vi "Open.vi"(8 "error in (no error)":errorcluster) -> (0 "error out":errorcluster, 3 "FPGA Refs":T1)   [LabVIEW 2017, in "Piezo Controller.lvlib"]
uses:
  Piezo Controller.lvlib
  FPGA Refs.ctl
  <instrlib>/_niInstr/FIFO Register Bus/v1/Host/niInstr FIFO Register Bus v1 Host.lvclass
  C:/Program Files (x86)/National Instruments/LabVIEW 2017/instr.lib/_niInstr/Instruction Framework/v1/Host/Instruction Target/niInstr Instruction Target v1 Host.lvclass
  <instrlib>/_niInstr/Instruction Framework/v1/Host/Instruction Framework Context/niInstr Instruction Framework Context v1 Host.lvclass
  <vilib>/FPGAPlugInAG/PCIe-7852R/niLvFpga_Open_PCIe-7852R.vi
  <vilib>/rvi/interface/common/dynamic/niFpgaDynamicAddResources.vi
  <instrlib>/_niInstr/Instruction Framework/v1/Host/Subsystem Map/Private/Lookup Single Context.vi
  <vilib>/rvi/interface/nirviOpenFPGA/nirviOpenFPGA.xnode
  Builds/Bitfile/vibratome_single_channel.lvbitx
  <instrlib>/_niInstr/Instruction Framework/v1/Host/Subsystem Map/niInstr Subsystem Map v1 Host.lvclass
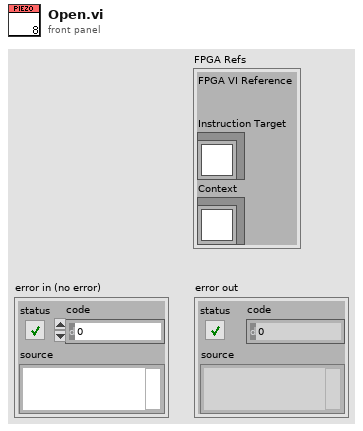
[diagram p1: front panel]
types:
  T1 = typedef "Piezo Controller.lvlib/FPGA Refs.ctl" = cluster{"FPGA VI Reference":refnum<k20>, "Instruction Target":refnum<class "niInstr FIFO Register Bus v1 Host.lvclass">, "Context":refnum<class "niInstr Instruction Framework Context v1 Host.lvclass">}
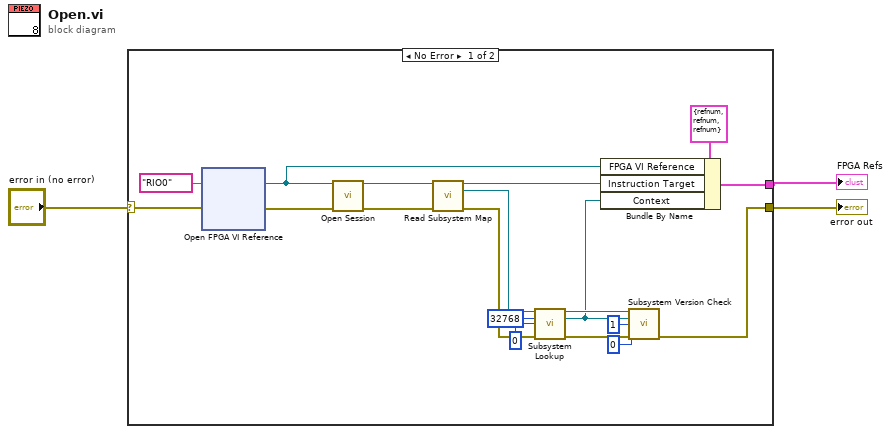
[diagram p0: block diagram]
diagram:
  n1 = case shown="No Error" "error in (no error)" {
    selector: "error in (no error)" -> [w5 w23]
    tunnel: [w6 _] -> w1
    tunnel: [w4 w23] -> w2
    frame No Error {
      n2 = xnode "Open FPGA VI Reference"("error in"=w5, "resource name"=tag "RIO0") -> ("FPGA VI Reference Out"=w10:refnum<k20>, "error out"=w22:errorcluster)
      n3 = call <instrlib>:"Open Session.vi"("fpga ref"=w10, "error in"=w22) -> ("session out"=w20:refnum<class "niInstr FIFO Register Bus v1 Host.lvclass">, "error out"=w21:errorcluster)  [unwired: 12 in]
      n4 = call <instrlib>:"Read Subsystem Map.vi"("instruction target in"=w20, "error in"=w21) -> ("instruction target out"=w9:refnum<class "niInstr FIFO Register Bus v1 Host.lvclass">, "subsystem map"=w14:refnum<class "niInstr Subsystem Map v1 Host.lvclass">, "error out"=w19:errorcluster)  [unwired: 11 in]
      n5 = call-poly <instrlib>:"Subsystem Lookup.vi"("subsystem map in"=w14, "UID"=u16 32768, "instance"=u8 0, "error in"=w19) -> ("subsystem map out"=w17:refnum<class "niInstr Subsystem Map v1 Host.lvclass">, "context"=w8:refnum<class "niInstr Instruction Framework Context v1 Host.lvclass">, "error out"=w18:errorcluster)  [unwired: 8 in, 1 out]
      n6 = Bundle By Name(cluster=T1 {"FPGA VI Reference"=refnum, "Instruction Target"=refnum, "Context"=refnum} ("output cluster"), "FPGA VI Reference"=w10, "Instruction Target"=w9, "Context"=w8) -> (w6:T1)
      n7 = call-dynamic "Subsystem Version Check.vi"("subsystem map in"=w17, "context"=w8, "version"=u16 1, "oldest compatible version"=u16 0, "error in"=w18) -> ("error out"=w4:errorcluster)  [unwired: 7 in, 3 out]
    }
    frame Error {
    }
  }
  "error out" <- w2
  "FPGA Refs" <- w1
